vi "Generate mounth year strings.vi"(7 "Dashes?":bool, 11 "seconds since 1904 (default 0 = now)":u32) -> (0 "mmdd":string, 3 "Month_year":string)   [LabVIEW 2012]
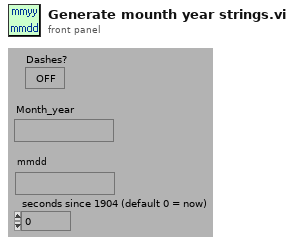
[diagram p1: front panel]
types:
  T1 = typedef "LVDateTimeRec.ctl" = cluster{"fractional second":dbl, "second":i32, "minute":i32, "hour":i32, "day of month":i32, "month":i32, "year":i32, "day of week":i32, "day of year":i32, "DST":i32}
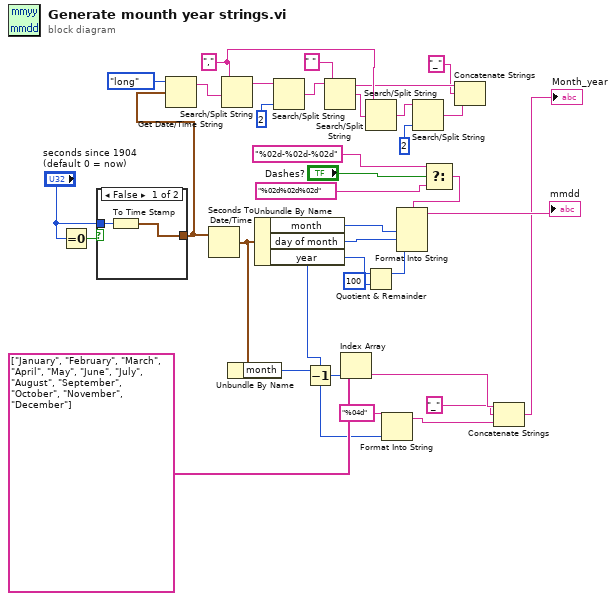
[diagram p0: block diagram]
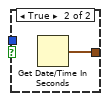
[diagram p2: hidden frame]
diagram:
  w27 = ","
  n1 = Equal To 0?(x="seconds since 1904 (default 0 = now)") -> (x = 0?=w22:bool)
  n2 = case shown="False" w22 {
    tunnel: [w36 w38] -> w17
    tunnel: "seconds since 1904 (default 0 = now)" -> [w37 _]
    frame False {
      n3 = To Time Stamp(1:w37) -> (0:w36:timestamp)
    }
    frame True {
      n4 = Get Date/Time In Seconds() -> (seconds since 1Jan1904=w38:timestamp)
    }
  }
  n5 = Get Date/Time String(date format (0)=enum16{"short", "long", "abbreviated"}."long", seconds (now)=w17) -> (date string=w35:string)  [unwired: 2 out]
  n6 = Seconds To Date/Time(time stamp (now)=w17) -> (date time rec=w11:T1)  [unwired: 1 out]
  n7 = Search/Split String(string=w35, search string/char (-)=w27) -> (match + rest of string=w33:string)  [unwired: 3 out]
  n8 = Unbundle By Name(w11) -> ("month"=w2:i32)
  n9 = Unbundle By Name(w11) -> ("month"=w20:i32, "day of month"=w19:i32, "year"=w8:i32)
  n10 = Search/Split String(string=w33, offset (0)=2) -> (match + rest of string=w32:string)  [unwired: 3 out]
  n11 = Decrement(x=w2) -> (x-1=w1:i32)
  n12 = Search/Split String(string=w32, search string/char (-)=" ") -> (substring before match=w24:string, match + rest of string=w29:string)  [unwired: 2 out]
  n13 = Index Array(array=string[] ["January", "February", "March", "April", "May", "June", "July", "August", "September", "October", "November", "December"], index=w1) -> (element=w6:string)
  n14 = Search/Split String(string=w29, search string/char (-)=w27) -> (match + rest of string=w26:string)  [unwired: 3 out]
  n15 = Quotient & Remainder(x=w8, y=100) -> (x-y*floor(x/y)=w10:i32)  [unwired: 1 out]
  n16 = Format Into String(format string="%04d", w8) -> (resulting string=w4:string)  [unwired: 2 in, 1 out]
  n17 = Search/Split String(string=w26, offset (0)=2) -> (match + rest of string=w30:string)  [unwired: 3 out]
  n18 = Select(t="%02d-%02d-%02d", s="Dashes?", f="%02d%02d%02d") -> (s? t:f=w15:string)
  n19 = Format Into String(format string=w15, w20, w19, w10) -> (resulting string=→"mmdd":string)  [unwired: 2 in, 1 out]
  n20 = Concatenate Strings(w24, "_" ("substring before char"), w30) -> ()  [unwired: 1 out]
  n21 = Concatenate Strings(w6, "_" ("substring before char"), w4) -> (→"Month_year":string)
